vi "Read Pixels and Copy to Display Image Array.vi"(0 "fpga interface in":refnum<k20>, 5 "display channel number":i32, 7 "serial channel display parameters":T4[](array[typedef]) {"RAW parameters"."bayer parameters"."blue gain" format="%_4g"; "RAW parameters"."bayer parameters"."green gain" format="%_4g"; "RAW parameters"."bayer parameters"."red gain" format="%_4g"; "RAW parameters"."bayer parameters"."algorithm" items=["Bilinear", "VNG"]; "RAW parameters"."bayer parameters"."pattern" items=["GB", "GR", "BG", "RG"]}, 9 "image metadata":T2, 11 "error in (no error)":errorcluster) -> (4 "fpga interface out":refnum<k20>, 6 "display image":T1, 8 "Pixel Data":u8[](array[numeric]), 15 "error out":errorcluster)   [LabVIEW 2025, in "Automotive Vision.lvclass"]
uses:
  Automotive Vision.lvclass
  deps/NI148X/Getting Started/Host/Common/GettingStarted_Common_148X_Host.lvlib
  <instrlib>/FlexRIO/CSI-2/v2/Common/Types/LLP Data Type.ctl
  <instrlib>/FlexRIO/CSI-2/v2/Common/NI CSI-2 API Common v2.lvlib
  <vilib>/vision/Image Controls.llb/IMAQ Image.ctl
  deps/NI148X/Getting Started/Host/Common/Types/Serial Channel Display Parameters.ctl
  deps/NI148X/Getting Started/FPGA/Common/Types/Image Metadata.ctl
  deps/NI148X/Getting Started/FPGA/Common/GettingStarted_Common_148X_FPGA.lvlib
  deps/NI148X/Getting Started/Host/Common/Types/RAW Interpretation for Display.ctl
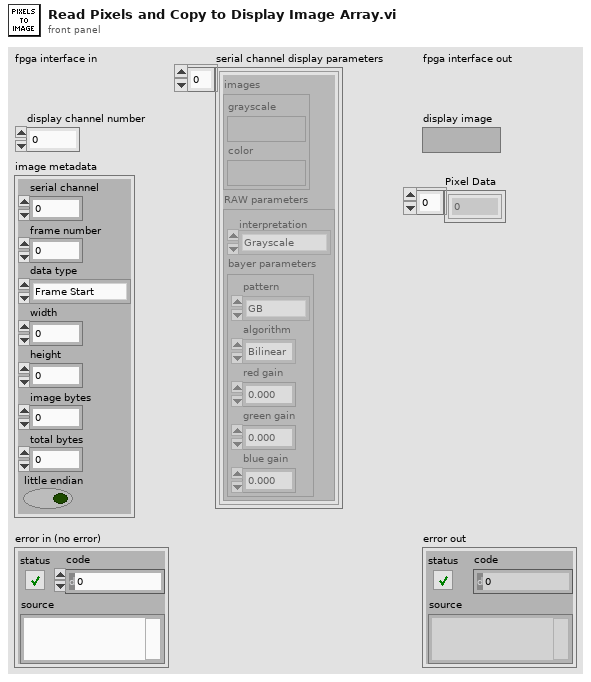
[diagram p1: front panel]
types:
  T1 = typedef "IMAQ Image.ctl" = refnum<image>
  T2 = typedef "GettingStarted_Common_148X_FPGA.lvlib/Image Metadata.ctl" = cluster{"serial channel":fxp<+,3,3>, "frame number":u16, "data type":T3, "width":u16, "height":u16, "image bytes":u32, "total bytes":u32, "little endian":bool}
  T3 = typedef "NI CSI-2 API Common v2.lvlib/LLP Data Type.ctl" = enum8{"Frame Start", "Frame End", "Line Start", "Line End", "End of Transmission", "Reserved 0", "Reserved 1", "Reserved 2", "Generic Short Packet 1", "Generic Short Packet 2", "Generic Short Packet 3", "Generic Short Packet 4", "Generic Short Packet 5", "Generic Short Packet 6", "Generic Short Packet 7", "Generic Short Packet 8", "Null", "Blanking Data", "Embedded 8-bit non Image Data", "Generic Long Packet 1", "Generic Long Packet 2", "Generic Long Packet 3", "Generic Long Packet 4", "Reserved 3", "YUV420 8-bit", "YUV420 10-bit", "Legacy YUV420 8-bit", "Reserved 4", "YUV420 8-bit Chroma Shifted", "YUV420 10-bit Chroma Shifted", "YUV422 8-bit", "YUV422 10-bit", "RGB444", "RGB555", "RGB565", "RGB666", "RGB888", "Reserved 5", "Reserved 6", "RAW 24", "RAW 6", "RAW 7", "RAW 8", "RAW 10", "RAW 12", "RAW 14", "RAW 16", "RAW 20", "User Defined 8-bit Data 1", "User Defined 8-bit Data 2", "User Defined 8-bit Data 3", "User Defined 8-bit Data 4", "User Defined 8-bit Data 5", "User Defined 8-bit Data 6", "User Defined 8-bit Data 7", "User Defined 8-bit Data 8", "USL Command", "Reserved 7", "Reserved 8", "Reserved 9", "Reserved 10", "Reserved 11", "Reserved 12", "LRTE EPD Spacer"}
  T4 = typedef "GettingStarted_Common_148X_Host.lvlib/Serial Channel Display Parameters.ctl" = cluster{"images":cluster{"grayscale":T1, "color":T1}, "RAW parameters":cluster{"interpretation":T5, "bayer parameters":cluster{"pattern":i32, "algorithm":i32, "red gain":dbl, "green gain":dbl, "blue gain":dbl}}}
  T5 = typedef "GettingStarted_Common_148X_Host.lvlib/RAW Interpretation for Display.ctl" = enum16{"Grayscale", "Bayer", "RGB", "YUV422", "YUV420", "Legacy YUV420"}
  T6 = cluster{"pattern":i32, "algorithm":i32, "red gain":dbl, "green gain":dbl, "blue gain":dbl}
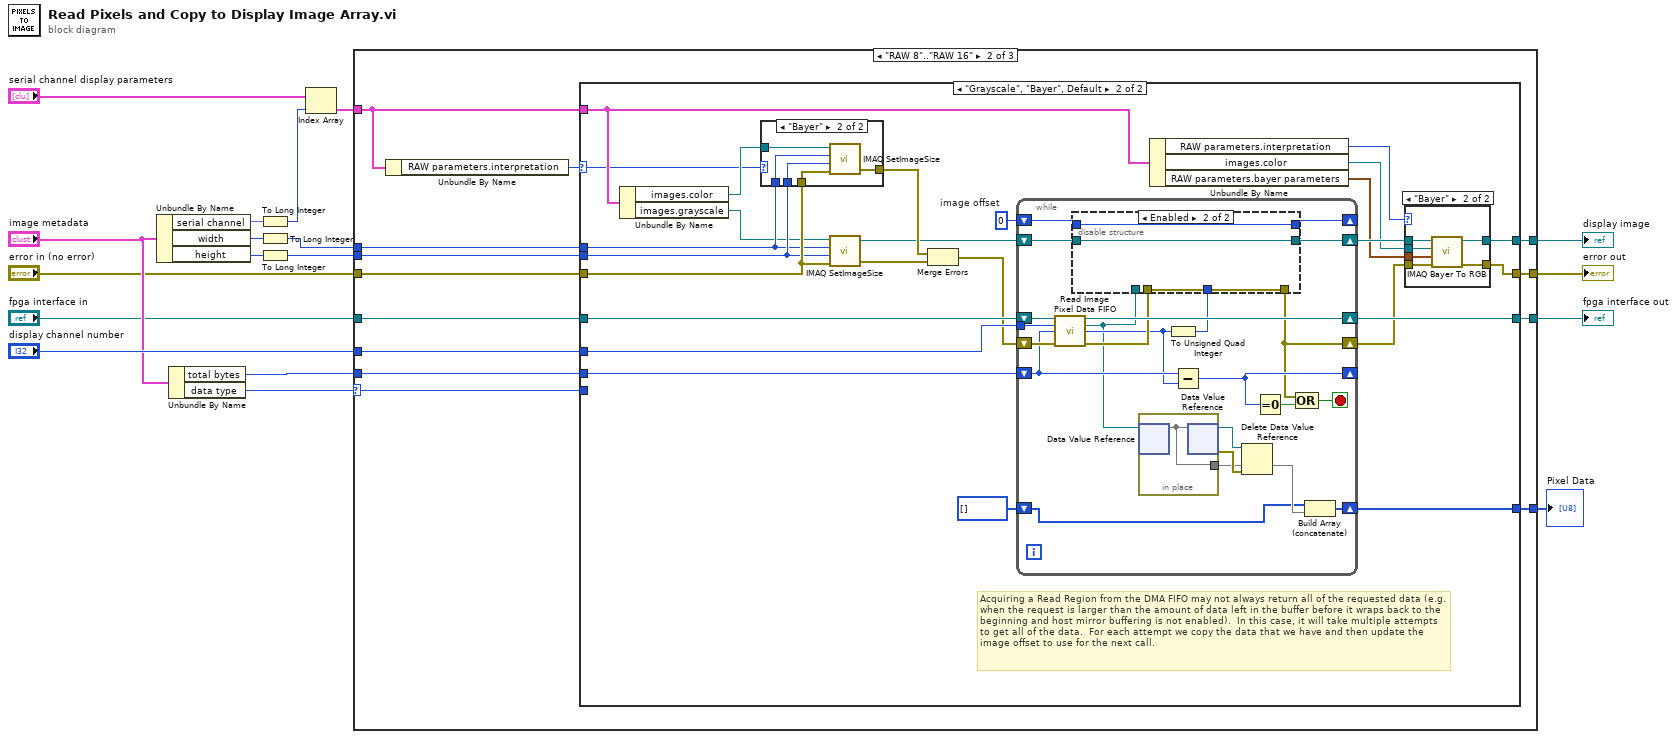
[diagram p0: block diagram]
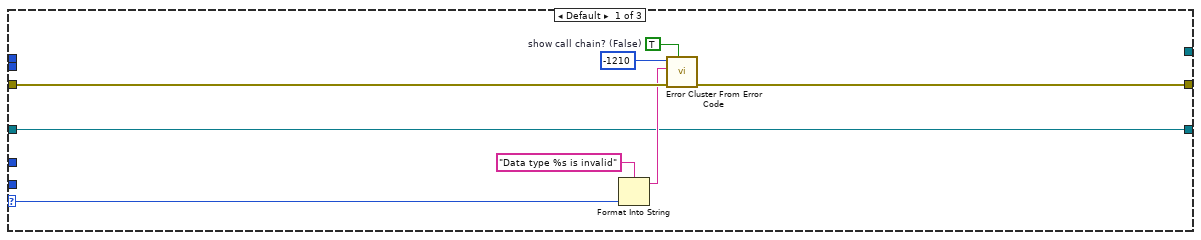
[diagram p2: hidden frame]
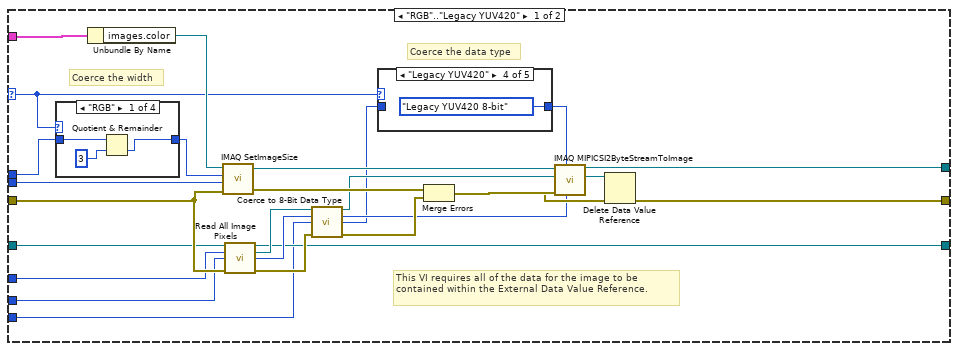
[diagram p3: hidden frame]
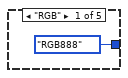
[diagram p4: hidden frame]
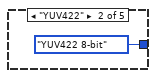
[diagram p5: hidden frame]
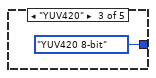
[diagram p6: hidden frame]
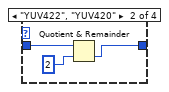
[diagram p8: hidden frame]
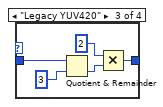
[diagram p9: hidden frame]
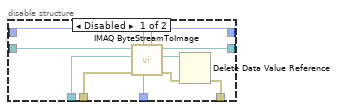
[diagram p12: hidden frame]
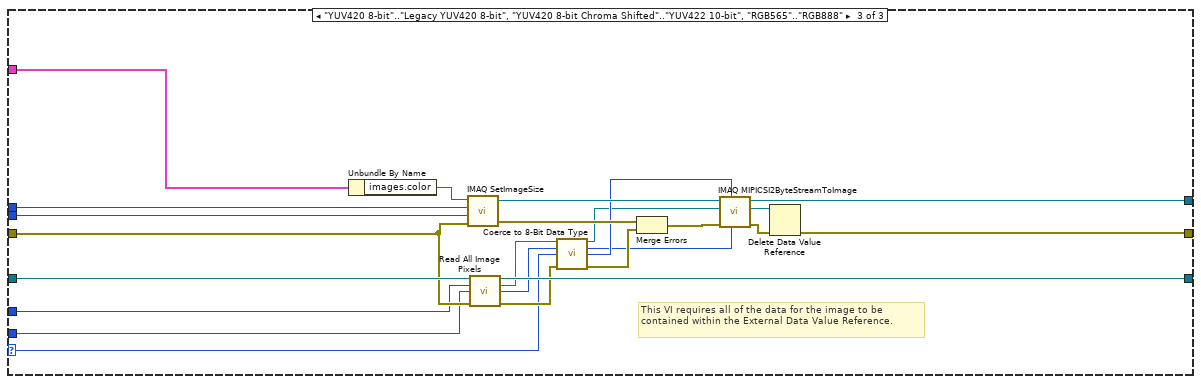
[diagram p14: hidden frame]
diagram:
  n1 = Unbundle By Name("image metadata") -> ("serial channel"=w14:fxp<+,3,3>, "width"=w10:u16, "height"=w11:u16)
  n2 = Unbundle By Name("image metadata") -> ("total bytes"=w17:u32, "data type"=w2:T3)
  n3 = To Long Integer(number=w14) -> (32bit integer=w12:i32)
  n4 = To Long Integer(number=w10) -> (32bit integer=w7:i32)
  n5 = To Long Integer(number=w11) -> (32bit integer=w8:i32)
  n6 = Index Array(array="serial channel display parameters", index=w12) -> (element=w4:T4)
  n7 = case shown="\"RAW 8\"..\"RAW 16\"" w2 {
    selector: w2 -> [w20 w28 w162]
    tunnel: w17 -> [_ w39 w172]
    tunnel: [w19 w38 w174] -> w16
    tunnel: "display channel number" -> [_ w37 w171]
    tunnel: "error in (no error)" -> [w24 w36 w175]
    tunnel: w8 -> [_ w35 w182]
    tunnel: w7 -> [_ w34 w181]
    tunnel: [_ w33 w170] -> w6
    tunnel: [w23 w32 w167] -> w5
    tunnel: w4 -> [_ w30 w179]
    tunnel: "fpga interface in" -> [w19 w31 w178]
    tunnel: [_ w27 _] -> w1
    frame Default {
      w25 = TRUE  # show call chain? (False)
      n8 = Format Into String(format string="Data type %s is invalid" ("error message (\"\")"), w20) -> (resulting string=w21:string)  [unwired: 2 in, 1 out]
      n9 = call <vilib>:"Error Cluster From Error Code.vi"("show call chain? (False)"=w25, "error in (no error)"=w24, "error message (\"\")"=w21, "error code (0)"=-1210) -> ("error out"=w23:errorcluster)  [unwired: 5 in]
    }
    frame "RAW 8".."RAW 16" {
      n10 = Unbundle By Name(w30) -> ("RAW parameters.interpretation"=w29:T5)
      n11 = case shown="\"Grayscale\", \"Bayer\", Default" w29 {
        selector: w29 -> [w42 w86]
        tunnel: w39 -> [w49 w108]
        tunnel: [w53 w106] -> w38
        tunnel: w37 -> [w48 w105]
        tunnel: w36 -> [w54 w104]
        tunnel: w35 -> [w45 w102]
        tunnel: w34 -> [w44 w101]
        tunnel: [w51 w98] -> w33
        tunnel: [w52 w96] -> w32
        tunnel: w30 -> [w47 w91]
        tunnel: w31 -> [w50 w90]
        tunnel: w28 -> [w46 _]
        tunnel: [_ w84] -> w27
        frame "RGB".."Legacy YUV420" {
          # "Coerce the data type"
          # "Coerce the width"
          # "This VI requires all of the data for the image to be contained within the External Data Value Reference."
          n12 = case shown="\"RGB\"" w42 {
            tunnel: w44 -> [w73 w76 w82 w83]
            tunnel: [w72 w75 w79 w83] -> w43
            frame "RGB" {
              n13 = Quotient & Remainder(x=w73, y=3) -> (floor(x/y)=w72:i32)  [unwired: 1 out]
            }
            frame "YUV422", "YUV420" {
              n14 = Quotient & Remainder(x=w76, y=2) -> (floor(x/y)=w75:i32)  [unwired: 1 out]
            }
            frame "Legacy YUV420" {
              n15 = Quotient & Remainder(x=w82, y=3) -> (floor(x/y)=w80:i32)  [unwired: 1 out]
              n16 = Multiply(x=2, y=w80) -> (x*y=w79:i32)
            }
            frame Default {
            }
          }
          n17 = Unbundle By Name(w47) -> ("images.color"=w66:T1)
          n18 = call "IMAQ SetImageSize"("error in (no error)"=w54, "Y Resolution"=w45, "X Resolution"=w43, "Image"=w66) -> ("error out"=w64:errorcluster, "Image Out"=w65:T1)  [unwired: 1 in]
          n19 = call "Read All Image Pixels.vi"("fpga inteface in"=w50, "display channel number"=w48, "image bytes"=w49, "error in (no error)"=w54) -> ("fpga interface out"=w53:refnum<k20>, "image pixel data region"=w59:refnum<data-value>, "elements in region"=w58:u32, "error out"=w60:errorcluster)  [unwired: 8 in]
          n20 = call "Coerce to 8-Bit Data Type.vi"("image pixel data region in"=w59, "image bytes in"=w58, "data type in"=w46, "error in (no error)"=w60) -> ("image pixel data region out"=w55:refnum<data-value>, "image bytes out"=w56:u32, "data type out"=w40:T3, "error out"=w57:errorcluster)  [unwired: 8 in]
          n21 = case shown="\"Legacy YUV420\"" w42 {
            tunnel: w40 -> [_ _ _ _ w71]
            tunnel: [LLP_Data_Type."RGB888" ("data type") LLP_Data_Type."YUV422 8-bit" ("data type") LLP_Data_Type."YUV420 8-bit" ("data type") LLP_Data_Type."Legacy YUV420 8-bit" ("data type") w71] -> w41
            frame "RGB" {
            }
            frame "YUV422" {
            }
            frame "YUV420" {
            }
            frame "Legacy YUV420" {
            }
            frame Default {
            }
          }
          n22 = Merge Errors(w64, w57) -> (w63:errorcluster)
          n23 = call "IMAQ MIPICSI2ByteStreamToImage"("Bytes to Copy"=w56, "Format"=w41, "error in (no error)"=w63, "Byte Stream In"=w55, "Image In"=w65) -> ("error out"=w62:errorcluster, "Byte Stream Out"=w61:refnum<data-value>, "Image Out"=w51:T1)  [unwired: 3 in, 1 out]
          n24 = Delete Data Value Reference(data value reference=w61, error in=w62) -> (error out=w52:errorcluster)  [unwired: 1 out]
        }
        frame "Grayscale", "Bayer", Default {
          w87 = u32 0  # image offset
          # "Acquiring a Read Region from the DMA FIFO may not always return all of the requested data (e.g. when the request is larger than the amount of data left in the buffer before it wraps back to the beginning and host mirror buffering is not enabled).  In this case, it will take multiple attempts to get all of the data.  For each attempt we copy the data that we have and then update the image offset to use for the next call."
          n25 = Unbundle By Name(w91) -> ("images.color"=w100:T1, "images.grayscale"=w95:T1)
          n26 = case shown="\"Bayer\"" w86 {
            tunnel: w104 -> [w109 w114]
            tunnel: [w109 w113] -> w103
            tunnel: w100 -> [_ w112]
            tunnel: w102 -> [_ w111]
            tunnel: w101 -> [_ w110]
            frame "Grayscale", Default {
            }
            frame "Bayer" {
              n27 = call "IMAQ SetImageSize"("error in (no error)"=w114, "Y Resolution"=w111, "X Resolution"=w110, "Image"=w112) -> ("error out"=w113:errorcluster)  [unwired: 1 in, 1 out]
            }
          }
          n28 = call "IMAQ SetImageSize"("error in (no error)"=w104, "Y Resolution"=w102, "X Resolution"=w101, "Image"=w95) -> ("error out"=w107:errorcluster, "Image Out"=w89:T1)  [unwired: 1 in]
          n29 = Merge Errors(w103, w107) -> (w88:errorcluster)
          n30 = while {
            tunnel: w105 -> [w134]
            shift-right: [w135] -> w106
            shift-left: w90 -> [w136]
            shift-right: [w123] -> w97
            shift-left: w88 -> [w133]
            shift-right: [w131] -> w99
            shift-left: w89 -> [w132]
            shift-right: [w126] -> _
            shift-left: w108 -> [w128]
            shift-right: [w122] -> _
            shift-left: w87 -> [w121]
            shift-right: [w117] -> w84
            shift-left: u8[] [] -> [w116]
            stop <- w124 stop-if-true
            n31 = call "Read Image Pixel Data FIFO.vi"("fpga inteface in"=w136, "display channel number"=w134, "number of elements"=w128, "error in (no error)"=w133) -> ("fpga interface out"=w135:refnum<k20>, "image pixel data region"=w115:refnum<data-value>, "elements in region"=w127:u32, "error out"=w130:errorcluster)  [unwired: 7 in, 1 out]
            n32 = in-place {
              in-place-border: [w150] -> w118
              n33 = in-place-dvr #1(w115) -> (w150:u8[])  [unwired: 1 out]
              n34 = in-place-dvr #1(w150) -> (w119:refnum<data-value>, w120:errorcluster)
            }
            n35 = To Unsigned Quad Integer(1:w127) -> (0:w129:u64)
            n36 = disable-structure shown="Enabled" {
              disable-tunnel: w132 -> [w146 w149]
              disable-tunnel: [w145 w149] -> w131
              disable-tunnel: w130 -> [w144 w148]
              disable-tunnel: w129 -> [w143 _]
              disable-tunnel: [w140 w148] -> w123
              disable-tunnel: [w139 w147] -> w122
              disable-tunnel: w121 -> [w138 w147]
              disable-tunnel: w115 -> [w137 _]
              frame Disabled {
                n37 = call "IMAQ ByteStreamToImage"("Bytes to Copy"=w143, "Image Byte Offset In"=w138, "error in (no error)"=w144, "Byte Stream In"=w137, "Image In"=w146) -> ("error out"=w141:errorcluster, "Byte Stream Out"=w142:refnum<data-value>, "Image Out"=w145:T1, "Image Byte Offset Out"=w139:u32)  [unwired: 2 in, 1 out]
                n38 = Delete Data Value Reference(data value reference=w142, error in=w141) -> (error out=w140:errorcluster)  [unwired: 1 out]
              }
              frame Enabled {
              }
            }
            n39 = Subtract(x=w128, y=w127) -> (x-y=w126:u32)
            n40 = Delete Data Value Reference(data value reference=w119, error in=w120) -> ()  [unwired: 2 out]
            n41 = Equal To 0?(x=w126) -> (x = 0?=w125:bool)
            n42 = Compound Arithmetic op=OR(w123, w125) -> (w124:bool)
            n43 = Build Array (concatenate)(w116, w118) -> (w117:u8[])
          }
          n44 = Unbundle By Name(w91) -> ("RAW parameters.interpretation"=w92:T5, "images.color"=w93:T1, "RAW parameters.bayer parameters"=w94:T6)
          n45 = case shown="\"Bayer\"" w92 {
            tunnel: w99 -> [w151 w158]
            tunnel: [w151 w157] -> w98
            tunnel: w97 -> [w152 w156]
            tunnel: [w152 w155] -> w96
            tunnel: w93 -> [_ w154]
            tunnel: w94 -> [_ w153]
            frame "Grayscale", Default {
            }
            frame "Bayer" {
              n46 = call "IMAQ Bayer To RGB"("error in (no error)"=w156, "Bayer Parameters"=w153, "Image Dst"=w154, "Image Src"=w158) -> ("error out"=w155:errorcluster, "Image Dst Out"=w157:T1)  [unwired: 6 in]
            }
          }
        }
      }
    }
    frame "YUV420 8-bit".."Legacy YUV420 8-bit", "YUV420 8-bit Chroma Shifted".."YUV422 10-bit", "RGB565".."RGB888" {
      # "This VI requires all of the data for the image to be contained within the External Data Value Reference."
      n47 = Unbundle By Name(w179) -> ("images.color"=w180:T1)
      n48 = call "IMAQ SetImageSize"("error in (no error)"=w175, "Y Resolution"=w182, "X Resolution"=w181, "Image"=w180) -> ("error out"=w176:errorcluster, "Image Out"=w177:T1)  [unwired: 1 in]
      n49 = call "Read All Image Pixels.vi"("fpga inteface in"=w178, "display channel number"=w171, "image bytes"=w172, "error in (no error)"=w175) -> ("fpga interface out"=w174:refnum<k20>, "image pixel data region"=w165:refnum<data-value>, "elements in region"=w164:u32, "error out"=w166:errorcluster)  [unwired: 8 in]
      n50 = call "Coerce to 8-Bit Data Type.vi"("image pixel data region in"=w165, "image bytes in"=w164, "data type in"=w162, "error in (no error)"=w166) -> ("image pixel data region out"=w159:refnum<data-value>, "image bytes out"=w160:u32, "data type out"=w161:T3, "error out"=w163:errorcluster)  [unwired: 8 in]
      n51 = Merge Errors(w176, w163) -> (w173:errorcluster)
      n52 = call "IMAQ MIPICSI2ByteStreamToImage"("Bytes to Copy"=w160, "Format"=w161, "error in (no error)"=w173, "Byte Stream In"=w159, "Image In"=w177) -> ("error out"=w169:errorcluster, "Byte Stream Out"=w168:refnum<data-value>, "Image Out"=w170:T1)  [unwired: 3 in, 1 out]
      n53 = Delete Data Value Reference(data value reference=w168, error in=w169) -> (error out=w167:errorcluster)  [unwired: 1 out]
    }
  }
  "display image" <- w6
  "fpga interface out" <- w16
  "error out" <- w5
  "Pixel Data" <- w1
